vi "chartPodSubPanel.vi"(11 "data":waveform(dbl)[](array[waveform])) -> (0 "vi reference":refnum<vi>, 3 "Waveform Chart - Dark":waveform(dbl)[](graph))   [LabVIEW 2017]
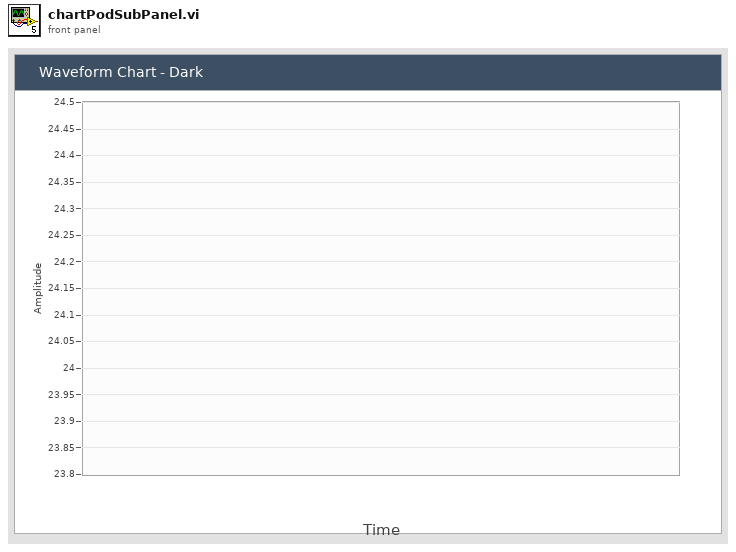
[diagram p1: front panel]
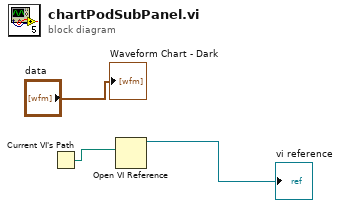
[diagram p0: block diagram]
diagram:
  n1 = Current VI's Path() -> (path=w2:path)
  n2 = Open VI Reference(vi path=w2) -> (vi reference=→"vi reference":refnum<vi>)  [unwired: 5 in, 1 out]
  "Waveform Chart - Dark" <- "data"
